vi "BuscarenInventario.vi"(8 "error in (no error)":errorcluster) -> (0 "error out":errorcluster, 3 "Array":T1[](array[typedef]))   [LabVIEW 2020, in "DataBaseSQLlite.lvlib"]
uses:
  DataBaseSQLlite.lvlib
  ProductInvenmtarytyppedef.ctl
  <vilib>/drjdpowell/SQLite Library/SQL Connection/Open (path).vi
  <vilib>/drjdpowell/SQLite Library/SQL Connection/Open (string).vi
  <vilib>/AdvancedString/Path To Command Line String.vi
  <vilib>/drjdpowell/SQLite Library/SQL Connection/Execute SQL (1D String).vi
  <vilib>/drjdpowell/SQLite Library/SQL Connection/Execute SQL (Single Integer).vi
  <vilib>/drjdpowell/SQLite Library/SQL Connection/Execute SQL (Single DBL).vi
  <vilib>/drjdpowell/SQLite Library/SQL Connection/Connection.lvclass
  <vilib>/drjdpowell/SQLite Library/SQLite.lvlib
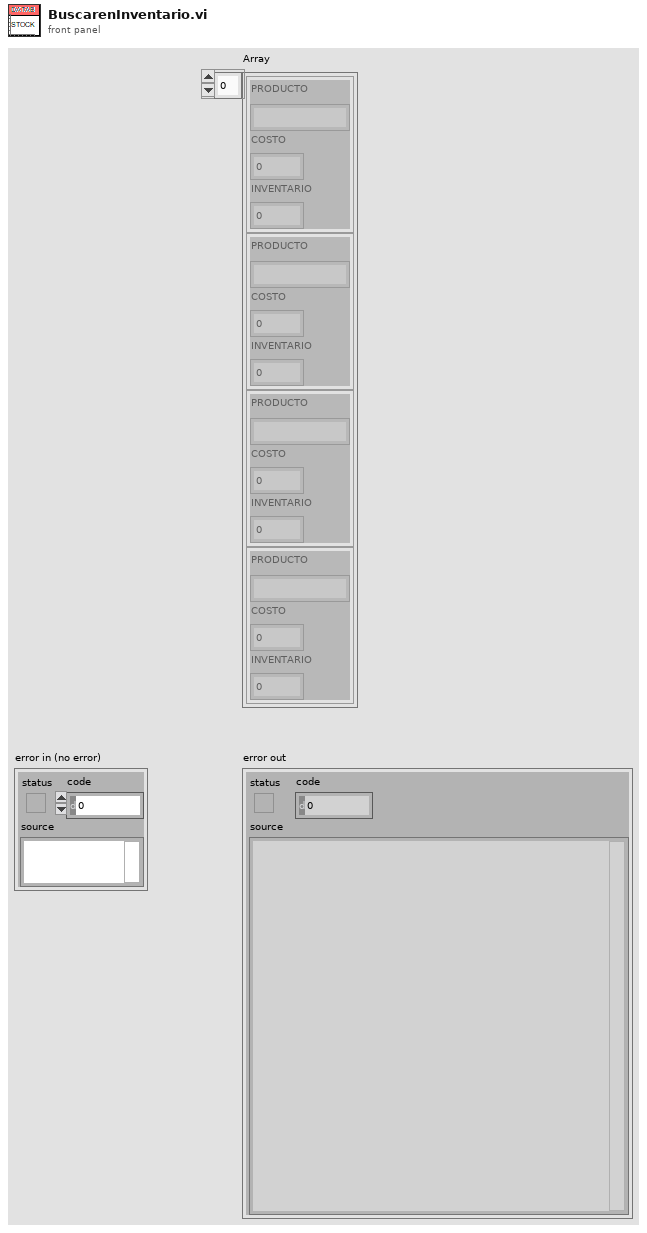
[diagram p1: front panel]
types:
  T1 = typedef "ProductInvenmtarytyppedef.ctl" = cluster{"PRODUCTO":string, "COSTO":dbl, "INVENTARIO":dbl}
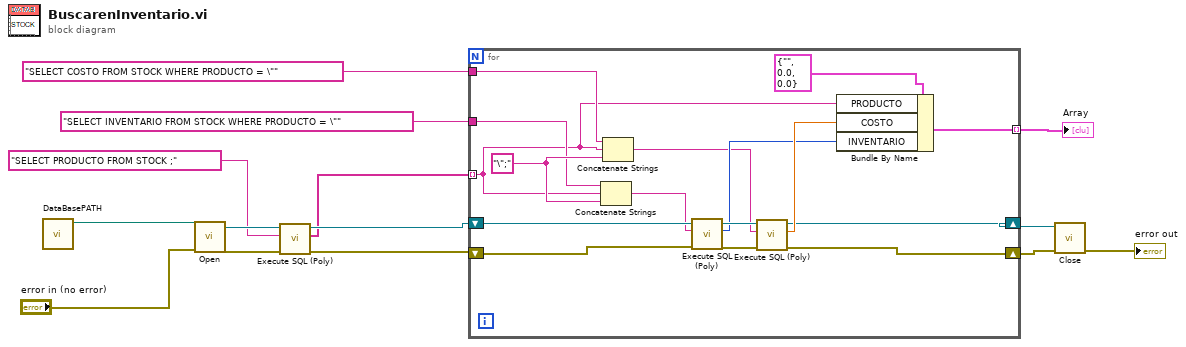
[diagram p0: block diagram]
diagram:
  n1 = call "DataBasePATH.vi"() -> ("DataBase path"=w14:path)  [unwired: 11 in]
  n2 = call-poly <vilib>:"Open.vi"("error in (no error)"="error in (no error)", "db file"=w14) -> ("error out"=w11:errorcluster, "SQLite Connection"=w12:refnum<class "Connection.lvclass">)  [unwired: 8 in]
  n3 = call-poly <vilib>:"Execute SQL (Poly).vi"("error in (no error)"=w11, "SQL"="SELECT PRODUCTO FROM STOCK ;", "SQLite Connection in"=w12) -> ("error out"=w6:errorcluster, "Result Set"=w7:string[], "SQLite Connection"=w8:refnum<class "Connection.lvclass">)  [unwired: 5 in, 1 out]
  n4 = for {
    shift-right: [w26] -> w9
    shift-left: w8 -> [w25]
    tunnel: w7 -> [w15] mode=indexing
    shift-right: [w22] -> w5
    shift-left: w6 -> [w23]
    tunnel: "SELECT INVENTARIO FROM STOCK WHERE PRODUCTO = \"" ("SQL") -> [w20]
    tunnel: "SELECT COSTO FROM STOCK WHERE PRODUCTO = \"" ("SQL") -> [w19]
    tunnel: [w17] -> w2 mode=indexing
    w21 = "\";"
    n5 = Concatenate Strings(w20, w15, w21) -> (w18:string)
    n6 = Concatenate Strings(w19, w15, w21) -> (w24:string)
    n7 = call-poly <vilib>:"Execute SQL (Poly).vi"("error in (no error)"=w23, "SQL"=w18, "SQLite Connection in"=w25) -> ("error out"=w29:errorcluster, "Result"=w27:i64, "SQLite Connection"=w30:refnum<class "Connection.lvclass">)  [unwired: 6 in]
    n8 = call-poly <vilib>:"Execute SQL (Poly).vi"("error in (no error)"=w29, "SQL"=w24, "SQLite Connection in"=w30) -> ("error out"=w22:errorcluster, "Result"=w28:dbl, "SQLite Connection"=w26:refnum<class "Connection.lvclass">)  [unwired: 6 in]
    n9 = Bundle By Name(cluster=T1 {"PRODUCTO"="", "COSTO"=0.0, "INVENTARIO"=0.0} ("Cluster"), "PRODUCTO"=w15, "COSTO"=w28, "INVENTARIO"=w27) -> (w17:T1)
  }
  "Array" <- w2
  n10 = call-dynamic "Close.vi"("error in (no error)"=w5, "SQLite Connection in"=w9) -> ("error out"=→"error out":errorcluster)  [unwired: 9 in]
